vi "LogInDialog.vi"() -> (3 "Active User":string)   [LabVIEW 2023]
uses:
  TypeDefs/Paths/UsersPath.ctl
  <vilib>/Utility/xml.llb/Write to XML File(string).vi
  <vilib>/Utility/xml.llb/Read From XML File(string).vi
panel:
  in  "New Username":string
  in  "Create Account Button":bool
  in  "LogIn Button":bool
  in  "Select Existing Account":u16(ring) items=["Ed van Bruggen", "Reed Cohen", "Andrea Pocar", "Thomas Pinto Franco", "Wesley Gillis", "Hannah Peltz Smalley", "Seth Thibado"]
  # "This is just a formality so that we can know who was using the\nsystem during acquisition. There is no personal or private \ninformation involved in creating an account."
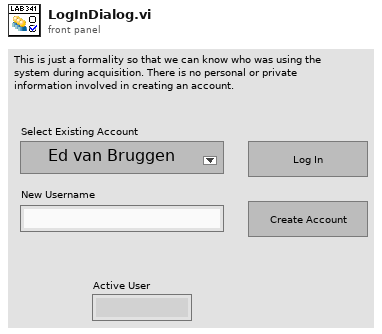
[diagram p1: front panel]
types:
  T1 = typedef "UsersPath.ctl" = path
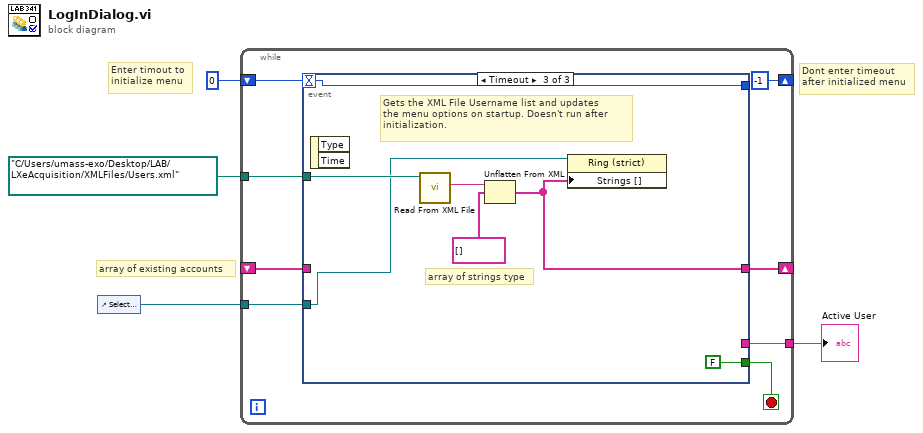
[diagram p0: block diagram]
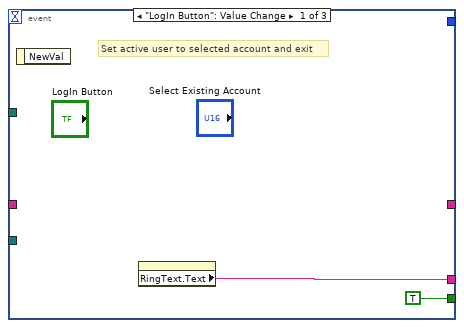
[diagram p2: hidden frame]
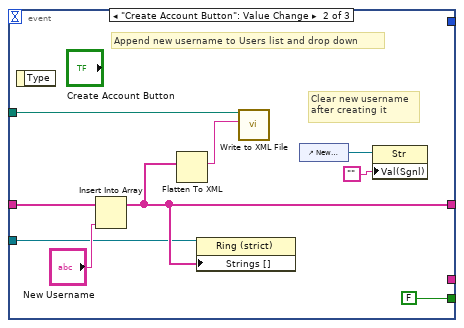
[diagram p3: hidden frame]
diagram:
  # "array of existing accounts"
  # "Enter timout to\ninitialize menu"
  # "Dont enter timeout\nafter initialized menu"
  n1 = control-ref of="Select Existing Account"() -> (w2:refnum<vi>)
  n2 = while {
    tunnel: T1 path "C:/Users/umass-exo/Desktop/LAB/LXeAcquisition/XMLFiles/Users.xml" ("XML File Path") -> [w12]
    shift-right: [w11] -> _
    shift-left: _ -> [w10]
    shift-right: [-1] -> _
    shift-left: 0 -> [w8]
    tunnel: [w7] -> w3
    tunnel: w2 -> [w5]
    stop <- w6 stop-if-true
    n3 = event shown="[2] Timeout" {
      selector: _ -> [_ _ _]
      dyn-events: _ -> [_ _ _]
      timeout: w8 -> [_ _ w30]
      tunnel: w10 -> [_ w23 _]
      tunnel: w12 -> [_ w21 w27]
      tunnel: [_ w19 w26] -> w11
      tunnel: [_ _ w30] -> _
      tunnel: [w14 _ _] -> w7
      tunnel: [TRUE FALSE FALSE] -> w6
      tunnel: w5 -> [_ w17 w24]
      event "LogIn Button": Value Change {
        # "Set active user to selected account and exit"
        n4 = event-data() -> ()  [unwired: 1 in, 1 out]
        n5 = property on="Select Existing Account" class="Ring (strict)"() -> ("RingText.Text"=w14:string)  [unwired: 2 in, 2 out]
      }
      event "Create Account Button": Value Change {
        # "Clear new username\nafter creating it"
        # "Append new username to Users list and drop down"
        n6 = event-data() -> ()  [unwired: 1 in, 1 out]
        n7 = Insert Into Array(array=w23, new element="New Username") -> (w19:string[])  [unwired: 1 in]
        n8 = Flatten To XML(6:w19) -> (2:w20:string)
        n9 = property on="Property Node" class="Ring (strict)"(reference=w17, "Strings []"=w19) -> ()  [unwired: 1 in, 2 out]
        n10 = call-poly <vilib>:"Write to XML File.vi"("XML Input"=w20, "XML File Path"=w21) -> ()  [unwired: 7 in, 3 out]
        n11 = control-ref of="New Username"() -> (w16:refnum<vi>)
        n12 = property class="Str"(reference=w16, "Val(Sgnl)"="") -> ()  [unwired: 1 in, 2 out]
      }
      event Timeout {
        # "array of strings type"
        # "Gets the XML File Username list and updates\nthe menu options on startup. Doesn't run after \ninitialization."
        n13 = event-data() -> ()  [unwired: 1 in, 2 out]
        n14 = call-poly <vilib>:"Read From XML File.vi"("XML File Path"=w27) -> ("XML Elements"=w29:string)  [unwired: 8 in, 2 out]
        n15 = Unflatten From XML(xml string=w29, type=string[] [] ("Strings []")) -> (value=w26:string[])  [unwired: 1 in, 1 out]
        n16 = property on="Property Node" class="Ring (strict)"(reference=w24, "Strings []"=w26) -> ()  [unwired: 1 in, 2 out]
      }
    }
  }
  "Active User" <- w3
